vi "SubMatrixB2.vi"(0 "BCluster":T1={"Target Field, T"=1.0, "Sweep rate, T/min"=1.0, "Time btw \npoints, sec"=1.0} {"Time btw \npoints, sec" format="%.2f"; "Sweep rate, T/min" min=0.0 max=1.0 step=0.01 format="%.4f"; "Target Field, T" min=-4.0 max=4.0 step=0.1 format="%.4f"}, 1 "Instruments":T3={"Oscillator"=TRUE, "Addr 1 lock-in"=TRUE, "Addr 1 lock-in oop"=TRUE, "Addr 2 lock-in"=FALSE, "Addr 2 lock-in oop"=FALSE, "Addr 3 lock-in"=FALSE, "Addr 3 lock-in oop"=FALSE, "Voltage (Vk1)"=FALSE, "Current (Ik1)"=TRUE, "Voltage (Vk2)"=FALSE, "Current (Ik2)"=FALSE, "Voltage (Vk3)"=FALSE, "Current (Ik3)"=FALSE, "Channel 1 (Vnano1)  "=FALSE, "Channel 2 (Vnano1b)"=FALSE, "Channel 1 (Vnano2)   "=FALSE, "Channel 2 (Vnano2b)"=FALSE, "Thermometer 1 (T1)"=TRUE, "Magnetic Field (B)"=TRUE, "Capacitance (C) and Loss (L)"=FALSE}, 2 "Settings":T2={"Ring 3"=1, "Ring 2"=4, "Fixed Current mkA"=0.5, "If yes, the current is:"=enum."Radio Selection 1", "Ressitance measurements?"=TRUE, "Commute DC current?"=FALSE} {"Ring 3" items=["1 kOhm", "10 kOhm", "100 kOhm", "1 Mohm", "10 mOhm"]; "Ring 2" items=["1 kOhm", "10 kOhm", "100 kOhm", "1 Mohm", "10 MOhm"]}, 3 "Custom Folder":string, 4 "Time Stamp":timestamp) -> ()   [LabVIEW 2017]
uses:
  <vilib>/Utility/file.llb/Write To Spreadsheet File (DBL).vi
panel:
  out "Vk2ini":dbl
  out "Communication":string
  out "Current":dbl
  out "Comments":string[](array[string])
  out "ArrayBoolian":bool[][](array[boolean])
  out "Delib Time delay":i32
  out "XY Graph":cluster{dbl[], dbl[]}(graph)={[1.0, 0.8, 0.6000000000000001, 0.4000000000000001, 0.20000000000000007, 5.551115123125783e-17, -0.19999999999999996, -0.39999999999999997, -0.6, -0.8, -1.0], [0.03352775, 0.056811, 0.03911575, 0.04330675, -0.02468015, 0.011641600000000002, 0.10151450000000001, 0.12386675000000001, 0.08288825000000001, -0.00186266, -0.038650000000000004]}
  out "array for data":dbl[](array[numeric])
  in  "Ring":u16(ring) caption="Y-axis:" items=["Vg", "Vk2", "Ik2", "Vnano1", "T1", "B", "cVk2", "cIk2", "cVnano1", "cT1", "cB"]
  out "Data file:":path
  # "Lock-in Amplifiers"
  # "Temperature"
  # "SourceMeters"
  # "Nanovoltmeters"
  # "Main"
  # "(not recommended, too slow)"
  # "Magnetic Field"
  # "Capacitance & Loss"
  # "(not recommended, too slow)"
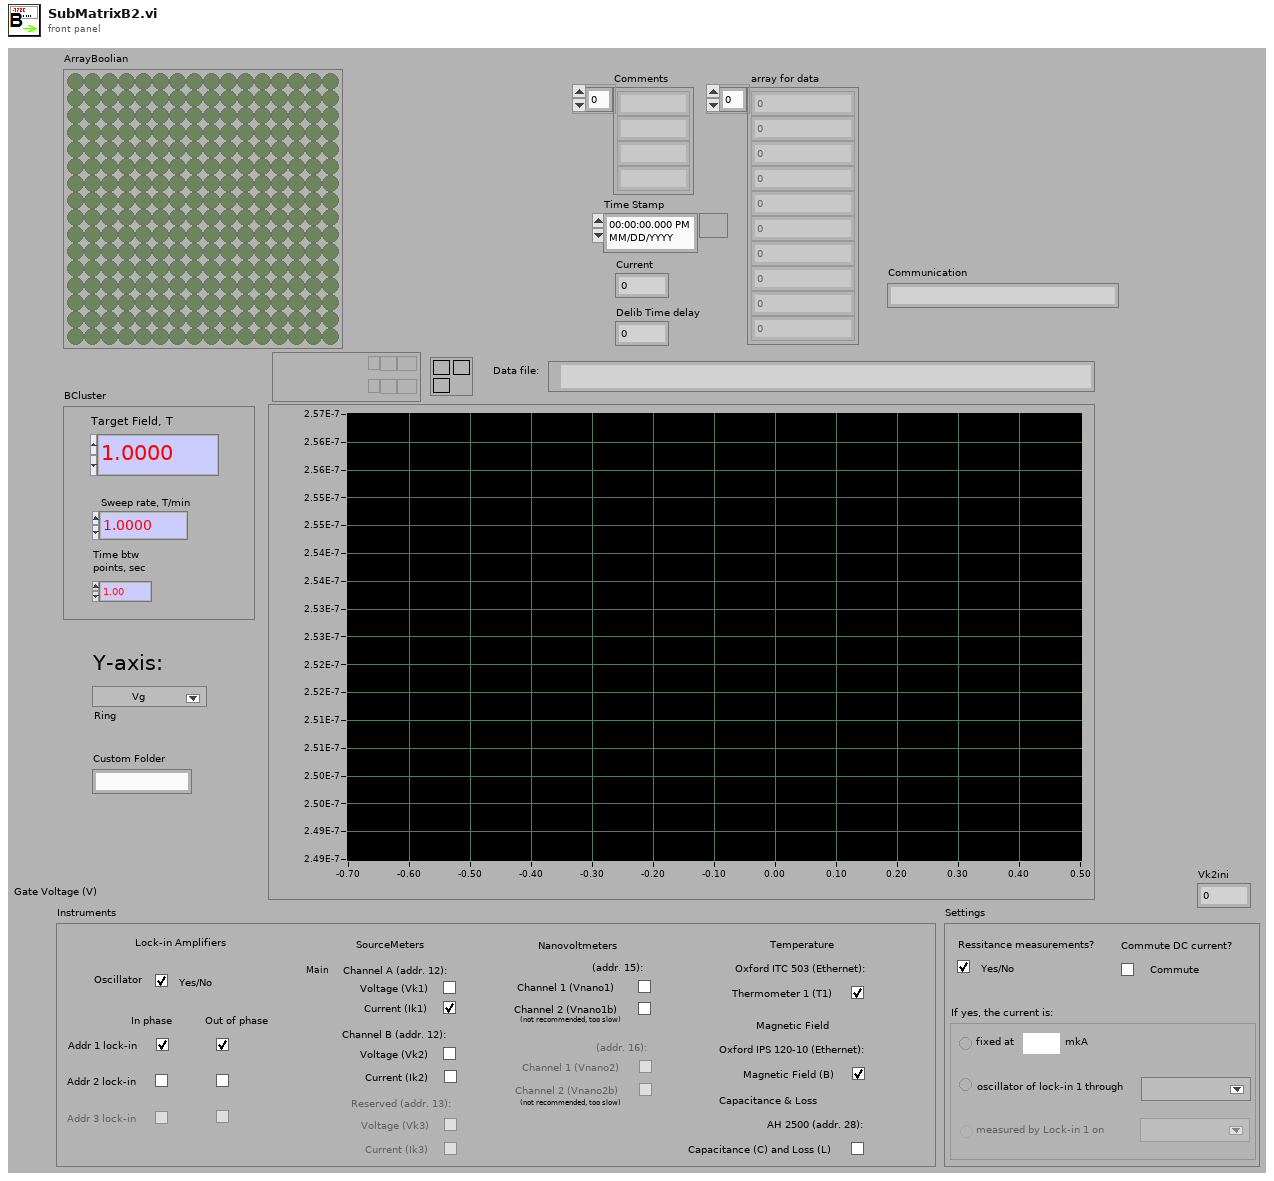
[diagram p1: front panel]
types:
  T1 = cluster{"Target Field, T":dbl, "Sweep rate, T/min":dbl, "Time btw \npoints, sec":dbl}
  T2 = cluster{"Ring 3":u16, "Ring 2":u16, "Fixed Current mkA":dbl, "If yes, the current is:":enum32{"Radio Selection 1", "Radio Selection 2", "Radio Selection 3"}, "Ressitance measurements?":bool, "Commute DC current?":bool}
  T3 = cluster{"Oscillator":bool, "Addr 1 lock-in":bool, "Addr 1 lock-in oop":bool, "Addr 2 lock-in":bool, "Addr 2 lock-in oop":bool, "Addr 3 lock-in":bool, "Addr 3 lock-in oop":bool, "Voltage (Vk1)":bool, "Current (Ik1)":bool, "Voltage (Vk2)":bool, "Current (Ik2)":bool, "Voltage (Vk3)":bool, "Current (Ik3)":bool, "Channel 1 (Vnano1)  ":bool, "Channel 2 (Vnano1b)":bool, "Channel 1 (Vnano2)   ":bool, "Channel 2 (Vnano2b)":bool, "Thermometer 1 (T1)":bool, "Magnetic Field (B)":bool, "Capacitance (C) and Loss (L)":bool}
  T4 = enum32{"Radio Selection 1", "Radio Selection 2", "Radio Selection 3"}
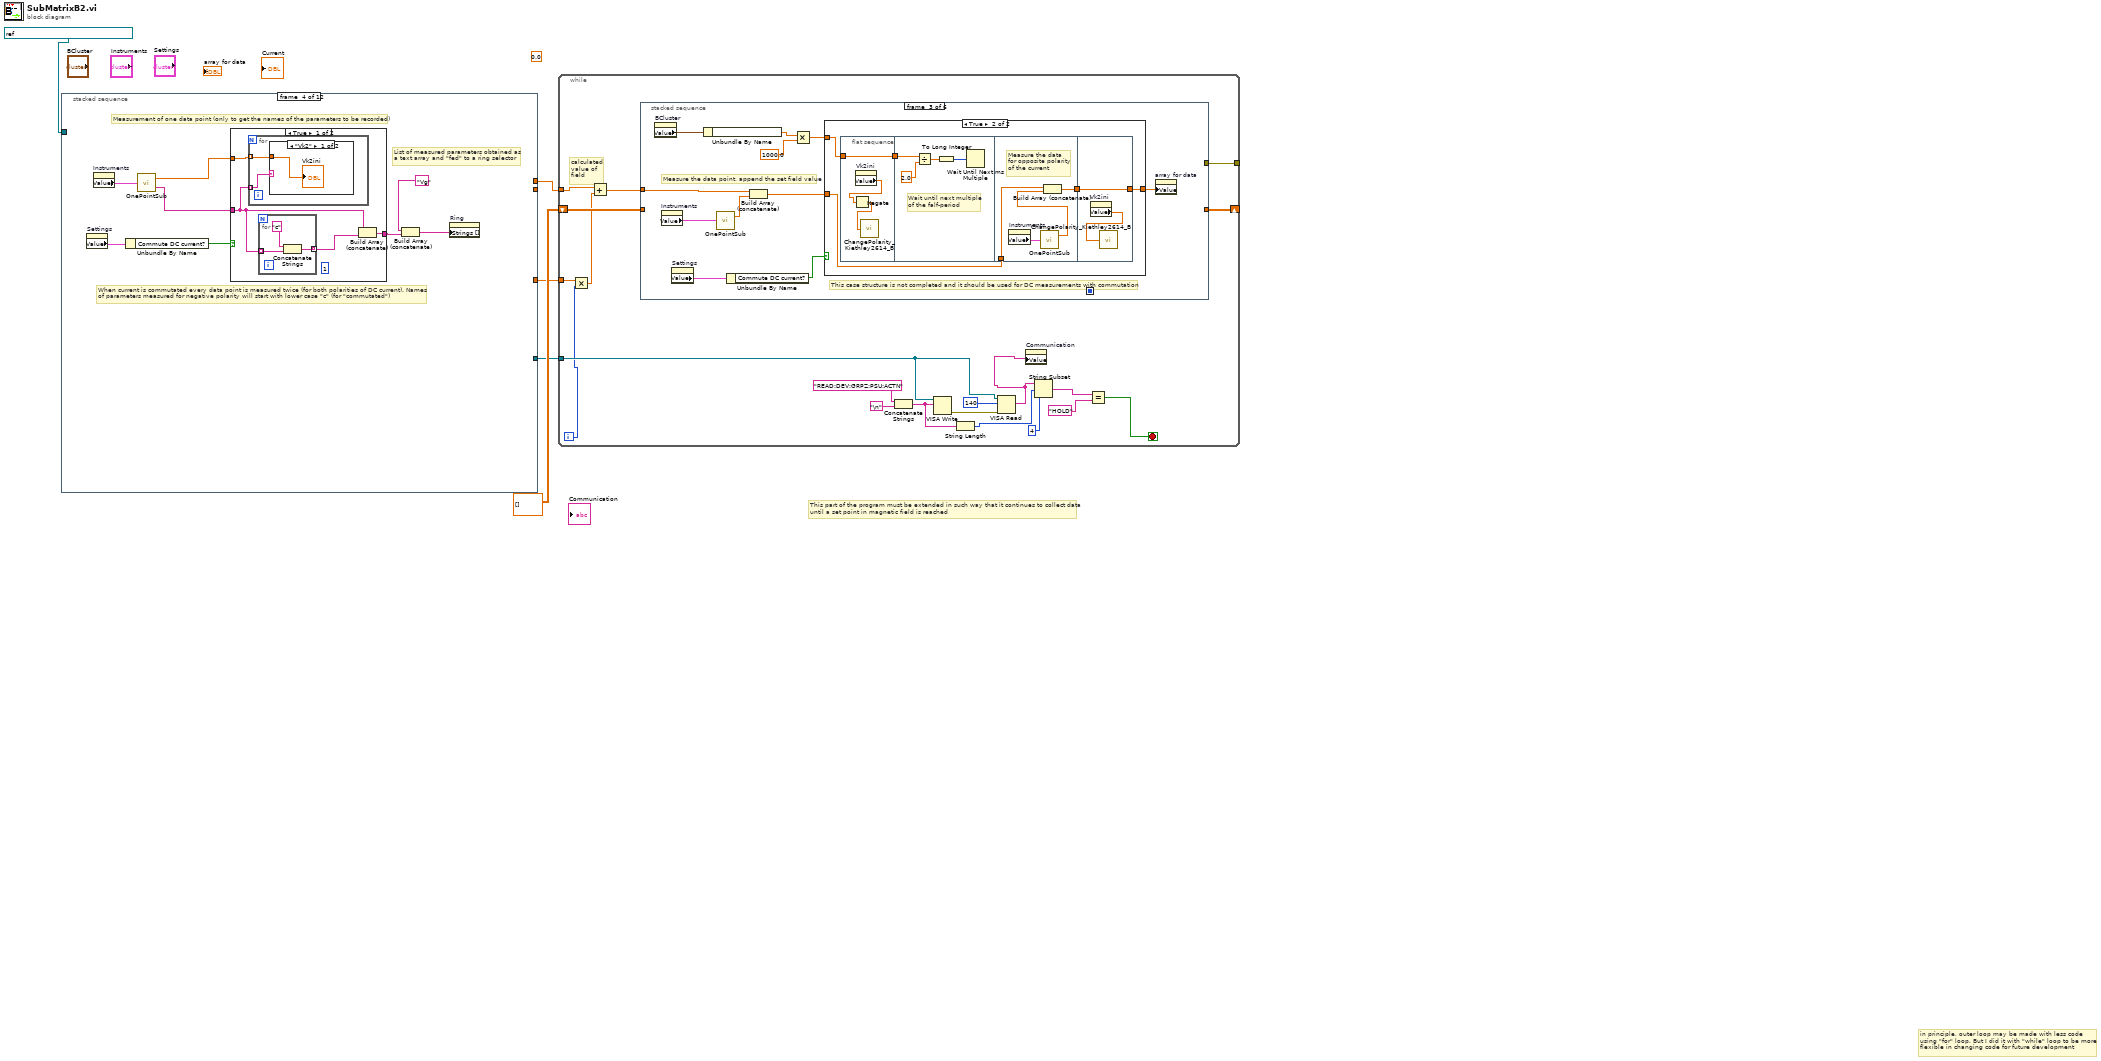
[diagram p0: block diagram]
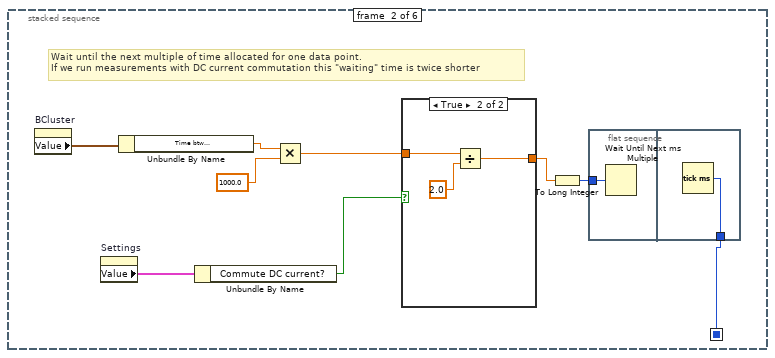
[diagram p3: hidden frame]
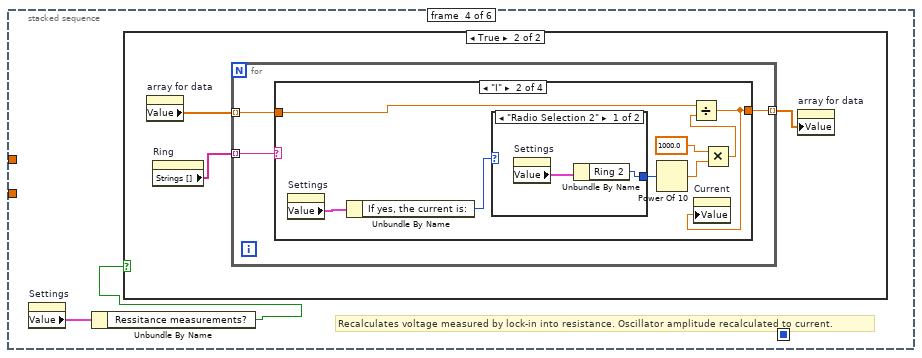
[diagram p6: hidden frame]
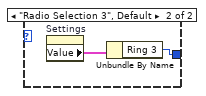
[diagram p9: hidden frame]
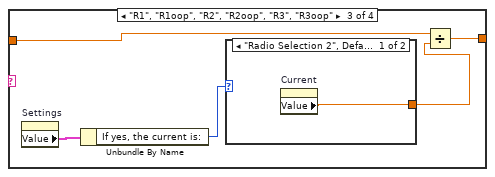
[diagram p10: hidden frame]
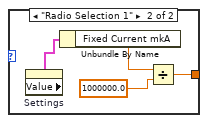
[diagram p11: hidden frame]
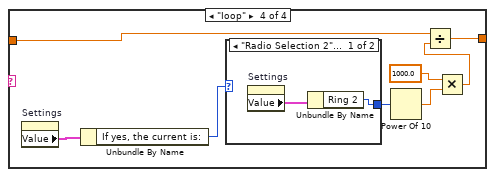
[diagram p12: hidden frame]
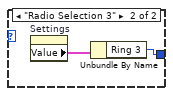
[diagram p13: hidden frame]
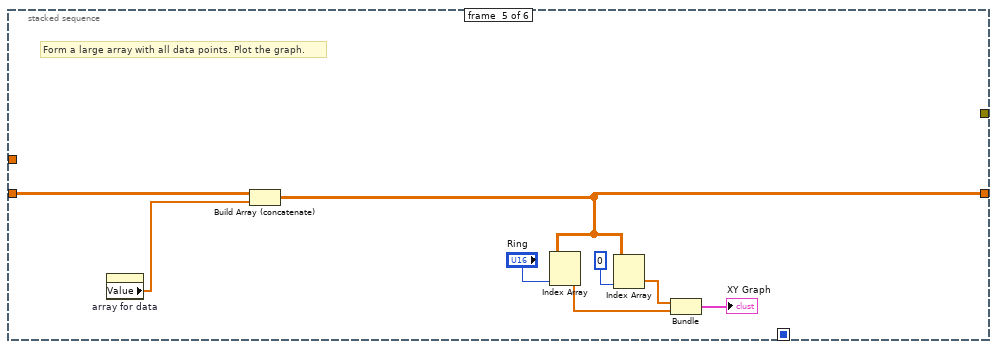
[diagram p14: hidden frame]
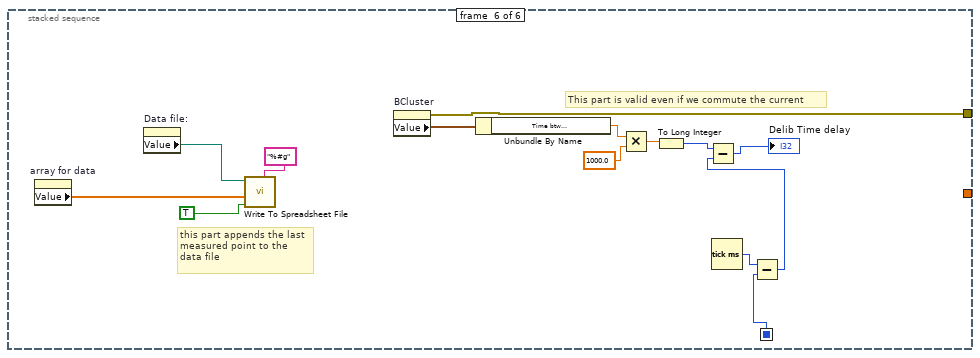
[diagram p15: hidden frame]
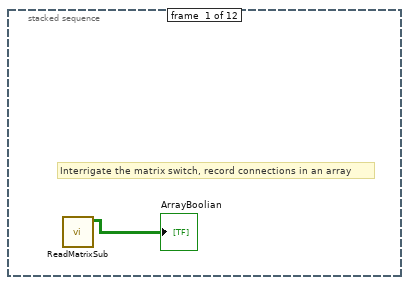
[diagram p16: hidden frame]
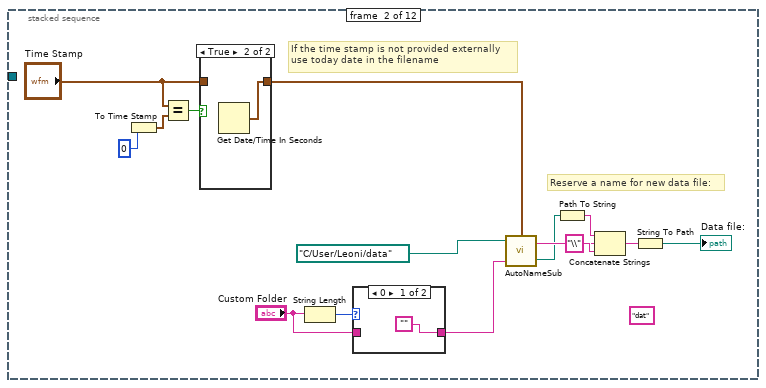
[diagram p17: hidden frame]
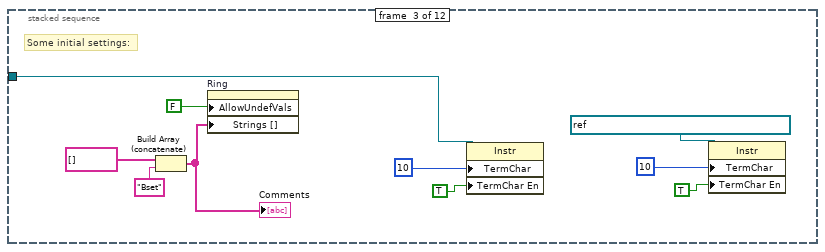
[diagram p20: hidden frame]
diagram:
  (unwired) 0.0
  # "This part of the program must be extended in such way that it continues to collect data\nuntil a set point in magnetic field is reached"
  # "in principle, outer loop may be made with less code\nusing \"for\" loop. But I did it with \"while\" loop to be more \nflexible in changing code for future development"
  n1 = stacked-sequence {
    tunnel: [_ _ _ _ _ _ _ _ _ w139 _ _] -> _
    tunnel: refnum<visa-resource-name> "TCPIP0::192.168.128.3::7020::SOCKET" ("VISA resource name") -> [_ _ w26 _ _ _ _ w100 _ w138 w174 w240]
    tunnel: [_ _ _ _ _ _ _ _ _ w138 _ _] -> w3
    tunnel: [_ _ _ _ _ _ _ _ _ w133 _ _] -> w2
    tunnel: [_ _ _ _ _ _ _ _ _ w132 _ _] -> w1
    frame #0 {
      # "Interrigate the matrix switch, record connections in an array"
      n2 = call "ReadMatrixSub.vi"() -> ("Array"=→"ArrayBoolian":bool[][])  [unwired: 9 in, 2 out]
    }
    frame #1 {
      (unwired) "dat"
      # "If the time stamp is not provided externally\nuse today date in the filename"
      # "Reserve a name for new data file:"
      n3 = To Time Stamp(1:0) -> (0:w10:timestamp)
      n4 = Equal?(x="Time Stamp", y=w10) -> (x = y?=w9:bool)
      n5 = case shown="True" w9 {
        tunnel: "Time Stamp" -> [w22 _]
        tunnel: [w22 w23] -> w7
        frame False {
        }
        frame True {
          n6 = Get Date/Time In Seconds() -> (seconds since 1Jan1904=w23:timestamp)
        }
      }
      n7 = String Length(string="Custom Folder") -> (length=w14:i32)
      n8 = case shown="0" w14 {
        tunnel: "Custom Folder" -> [_ w25]
        tunnel: ["" w25] -> w12
        frame 0 {
        }
        frame 1, Default {
        }
      }
      n9 = call "AutoNameSub.vi"("Time Stamp"=w7, "Custom Folder"=w12, "User Data Folder"=path "C:/User/Leoni/data") -> ("created path"=w20:path, "String"=w21:string)  [unwired: 1 in]
      n10 = Path To String(path=w20) -> (string=w15:string)
      n11 = Concatenate Strings(w15, "\\", w21) -> (w17:string)
      n12 = String To Path(string=w17) -> (path=→"Data file:":path)
    }
    frame #2 {
      # "Some initial settings:"
      n13 = Build Array (concatenate)(string[] [], "Bset") -> (w27:string[])
      "Comments" <- w27
      n14 = property on="Ring" class="Ring (strict)"("AllowUndefVals"=FALSE, "Strings []"=w27) -> ()  [unwired: 2 in, 2 out]
      n15 = property class="Instr"(reference=w26, "TermChar"=10, "TermChar En"=TRUE) -> ()  [unwired: 1 in, 2 out]
      n16 = property class="Instr"(reference=refnum<visa-resource-name> "TCPIP0::192.168.128.2::7020::SOCKET" ("VISA resource name"), "TermChar"=10, "TermChar En"=TRUE) -> ()  [unwired: 1 in, 2 out]
    }
    frame #3 {
      # "List of measured parameters obtained as \na text array and \"fed\" to a ring selector"
      # "When current is commutated every data point is measured twice (for both polarities of DC current). Names \nof parameters measured for negative polarity will start with lower case \"c\" (for \"commutated\")"
      # "Measurement of one data point (only to get the names of the parameters to be recorded)"
      n17 = property on="Settings" class="Clust (strict)"() -> ("Value"=w42:T2)  [unwired: 2 in, 2 out]
      n18 = property on="Instruments" class="Clust (strict)"() -> ("Value"=w40:T3)  [unwired: 2 in, 2 out]
      n19 = Unbundle By Name(w42) -> ("Commute DC current?"=w43:bool)
      n20 = call "OnePointSub.vi"("cluster"=w40) -> ("TextArray"=w41:string[], "Array"=w36:dbl[])  [unwired: 2 in]
      n21 = case shown="True" w43 {
        tunnel: w41 -> [w46 w54]
        tunnel: [w47 w54] -> w39
        tunnel: w36 -> [w45 _]
        frame True {
          (unwired) 1
          n22 = for {
            tunnel: w46 -> [w49] mode=indexing
            tunnel: w45 -> [w48] mode=indexing
            n23 = case shown="\"Vk2\"" w49 {
              tunnel: w48 -> [w50 _]
              frame "Vk2" {
                "Vk2ini" <- w50
              }
              frame Default {
              }
            }
          }
          n24 = for {
            tunnel: [w53] -> w44 mode=indexing
            tunnel: w46 -> [w51] mode=indexing
            n25 = Concatenate Strings("c", w51) -> (w53:string)
          }
          n26 = Build Array (concatenate)(w46, w44) -> (w47:string[])
        }
        frame False {
        }
      }
      n27 = Build Array (concatenate)("Vg", w39) -> (w37:string[])
      n28 = property on="Ring" class="Ring (strict)"("Strings []"=w37) -> ()  [unwired: 2 in, 2 out]
    }
    frame #4 {
      # "If resistance is not something that we are interested in, then replace \"R\" with \"V\" in all strings"
      n29 = property on="Settings" class="Clust (strict)"() -> ("Value"=w55:T2)  [unwired: 2 in, 2 out]
      n30 = Unbundle By Name(w55) -> ("Ressitance measurements?"=w56:bool)
      n31 = case shown="False" w56 {
        frame True {
        }
        frame False {
          n32 = property on="Ring" class="Ring (strict)"() -> ("Strings []"=w58:string[])  [unwired: 2 in, 2 out]
          n33 = for {
            tunnel: w58 -> [w61] mode=indexing
            tunnel: [w59] -> w57 mode=indexing
            n34 = String Subset(string=w61, length (rest)=1) -> (substring=w63:string)  [unwired: 1 in]
            n35 = Equal?(x=w63, y="R") -> (x = y?=w62:bool)
            n36 = case shown="True" w62 {
              tunnel: w61 -> [w65 w69]
              tunnel: [w65 w66] -> w59
              frame False {
              }
              frame True {
                n37 = Replace Substring(2:1, 4:"V", 5:w69) -> (1:w66:string)  [unwired: 1 in, 1 out]
              }
            }
          }
          n38 = property on="Ring" class="Ring (strict)"("Strings []"=w57) -> ()  [unwired: 2 in, 2 out]
        }
      }
    }
    frame #5 {
      # "This part makes comment line for the \ndata file. Comments are very useful for\ndouble checking that connections are \ncorrect when the data file is opened\nin Origin."
      # "Check how the oscillator is wired to the matrix switch and record connection as a comment"
      n39 = property on="Instruments" class="Clust (strict)"() -> ("Value"=w72:T3)  [unwired: 2 in, 2 out]
      n40 = property on="Comments" class="Arr (strict)"() -> ("Value"=w71:string[])  [unwired: 2 in, 2 out]
      n41 = Unbundle By Name(w72) -> ("Oscillator"=w73:bool)
      n42 = case shown="True" w73 {
        tunnel: [w74 w77] -> w70
        tunnel: w71 -> [w74 w76]
        frame False {
          # "we are not measuring oscillator from\nlock-in (address 1)"
        }
        frame True {
          (unwired) "I"
          # "This subVI takes the matrix column # (instrument\nconnection point) as an argument and finds the raw\n# (contact) to which the instrument is connected"
          # "we are  measuring oscillator"
          n43 = property on="ArrayBoolian" class="Arr (strict)"() -> ("Value"=w80:bool[][])  [unwired: 2 in, 2 out]
          n44 = GPIB Clear(3:"1") -> ()  [unwired: 1 in, 2 out]
          n45 = call "FindInstrConnect.vi"("Column #"=1, "ArrayBoolian"=w80) -> ("String"=w81:string)  [unwired: 1 in, 2 out]
          n46 = call "FindInstrConnect.vi"("Column #"=0, "ArrayBoolian"=w80) -> ("String"=w78:string)  [unwired: 1 in, 2 out]
          n47 = Concatenate Strings(w78, "-", w81) -> (w75:string)
          n48 = Build Array (concatenate)(w76, w75) -> (w77:string[])
        }
      }
      n49 = property on="Comments" class="Arr (strict)"("Value"=w70) -> ()  [unwired: 2 in, 2 out]
    }
    frame #6 {
      # "Check how the input of Lock-in 1 is wired the the matrix switch and record connection as a comment"
      n50 = property on="Instruments" class="Clust (strict)"() -> ("Value"=w87:T3)  [unwired: 2 in, 2 out]
      n51 = property on="Comments" class="Arr (strict)"() -> ("Value"=w86:string[])  [unwired: 2 in, 2 out]
      n52 = Unbundle By Name(w87) -> ("Addr 1 lock-in"=w88:bool)
      n53 = case shown="True" w88 {
        tunnel: [w89 w92] -> w85
        tunnel: w86 -> [w89 w91]
        frame False {
          # "we are not measuring oscillator from\nlock-in (address 1)"
        }
        frame True {
          (unwired) "I"
          # "This subVI takes the matrix column # (instrument\nconnection point) as an argument and finds the raw\n# (contact) to which the instrument is connected"
          # "we are  measuring Lock-In 1"
          n54 = property on="ArrayBoolian" class="Arr (strict)"() -> ("Value"=w95:bool[][])  [unwired: 2 in, 2 out]
          n55 = GPIB Clear(3:"1") -> ()  [unwired: 1 in, 2 out]
          n56 = call "FindInstrConnect.vi"("Column #"=3, "ArrayBoolian"=w95) -> ("String"=w96:string)  [unwired: 1 in, 2 out]
          n57 = call "FindInstrConnect.vi"("Column #"=2, "ArrayBoolian"=w95) -> ("String"=w93:string)  [unwired: 1 in, 2 out]
          n58 = Concatenate Strings(w93, "-", w96) -> (w90:string)
          n59 = Build Array (concatenate)(w91, w90) -> (w92:string[])
        }
      }
      n60 = property on="Comments" class="Arr (strict)"("Value"=w85) -> ()  [unwired: 2 in, 2 out]
    }
    frame #7 {
      n61 = while {
        tunnel: w100 -> [w110]
        stop <- w103 stop-if-true
        n62 = Wait (ms)(milliseconds to wait=500) -> ()  [unwired: 1 out]
        n63 = Concatenate Strings("READ:DEV:GRPZ:PSU:ACTN" ("string"), "\n") -> (w107:string)
        n64 = VISA Write(VISA resource name=w110, write buffer=w107) -> (error out=w113:errorcluster)  [unwired: 1 in, 2 out]
        n65 = String Length(string=w107) -> (length=w106:i32)
        n66 = VISA Read(VISA resource name=w110, byte count=140, error in (no error)=w113) -> (read buffer=w101:string)  [unwired: 3 out]
        n67 = property on="Communication" class="Str"("Value"=w101) -> ()  [unwired: 2 in, 2 out]
        n68 = String Subset(string=w101, offset (0)=w106, length (rest)=4) -> (substring=w105:string)
        n69 = Equal?(x=w105, y="HOLD") -> (x = y?=w103:bool)
      }
    }
    frame #8 {
      w122 = "\r"
      w121 = "\n"
      # "Both lines are recorded into\nthe data file."
      # "This part converts string array with the names of measured parameters into the line of text separated by TABs. The resulting string is\nrecorded as the first line of the data file. The second line is comments with information about conections of the instruments to particular contacts."
      n70 = property on="Ring" class="Ring (strict)"() -> ("Strings []"=w115:string[])  [unwired: 2 in, 2 out]
      n71 = property on="Comments" class="Arr (strict)"() -> ("Value"=w120:string[])  [unwired: 2 in, 2 out]
      n72 = for {
        tunnel: w115 -> [w130] mode=indexing
        shift-right: [w128] -> w118
        shift-left: "" -> [w129]
        n73 = Concatenate Strings(w129, w130, "\t") -> (w128:string)
      }
      n74 = for {
        tunnel: w120 -> [w126] mode=indexing
        shift-right: [w124] -> w123
        shift-left: "" -> [w125]
        n75 = Concatenate Strings(w125, w126, "\t") -> (w124:string)
      }
      n76 = Concatenate Strings(w118, w122, w121, w122, w121, w123, w122, w121) -> (w116:string)
      n77 = property on="Data file:" class="Path"() -> ("Value"=w114:path)  [unwired: 2 in, 2 out]
      n78 = Write to Text File(file (use dialog)=w114, text=w116) -> ()  [unwired: 2 in, 3 out]
    }
    frame #9 {
      # "Step"
      # "Read real field (persistant, if in persistance mode)"
      # "Then the table is made with all values\nof the gate voltage to be measured"
      # "rounding to 0.01 T"
      # "This part reads the status and current settings of the magnet"
      n79 = property on="BCluster" class="Clust (strict)"() -> ("Value"=w169:T1)  [unwired: 2 in, 2 out]
      n80 = Concatenate Strings("READ:DEV:GRPZ:PSU:SIG:PFLD" ("string"), "\n") -> (w159:string)
      n81 = VISA Write(VISA resource name=w138, write buffer=w159) -> (error out=w165:errorcluster)  [unwired: 1 in, 2 out]
      n82 = String Length(string=w159) -> (length=w160:i32)
      n83 = Unbundle By Name(w169) -> ("Target Field, T"=w137:dbl, "Sweep rate, T/min"=w142:dbl, "Time btw \npoints, sec"=w168:dbl)
      n84 = Number To Fractional String(number=w142) -> (F-format string=w148:string)  [unwired: 3 in]
      n85 = Concatenate Strings("SET:DEV:GRPZ:PSU:SIG:RFST:" ("string"), w148) -> (w143:string)
      n86 = VISA Read(VISA resource name=w138, byte count=140, error in (no error)=w165) -> (read buffer=w161:string)  [unwired: 3 out]
      n87 = Concatenate Strings(w143, "\n") -> (w144:string)
      n88 = Multiply(x=w142, y=w168) -> (x*y=w167:dbl)
      n89 = String Subset(string=w161, offset (0)=w160) -> (substring=w158:string)  [unwired: 1 in]
      n90 = Divide(x=w167, y=60.0) -> (x/y=w134:dbl)
      n91 = VISA Write(VISA resource name=w138, write buffer=w144) -> (error out=w147:errorcluster)  [unwired: 1 in, 2 out]
      n92 = Fract/Exp String To Number(string=w158) -> (number=w157:dbl)  [unwired: 3 in, 1 out]
      n93 = VISA Read(VISA resource name=w138, byte count=140, error in (no error)=w147) -> (read buffer=w140:string)  [unwired: 3 out]
      n94 = Number To Fractional String(number=w157, width (-)=4, precision (6)=2) -> (F-format string=w170:string)  [unwired: 1 in]
      n95 = Fract/Exp String To Number(string=w170) -> (number=w133:dbl)  [unwired: 3 in, 1 out]
      n96 = Number To Fractional String(number=w133) -> (F-format string=w155:string)  [unwired: 3 in]
      n97 = Concatenate Strings("SET:DEV:GRPZ:PSU:SIG:FSET:" ("string"), w155) -> (w150:string)
      n98 = Concatenate Strings(w150, "\n") -> (w151:string)
      n99 = VISA Write(VISA resource name=w138, write buffer=w151) -> (error out=w154:errorcluster)  [unwired: 1 in, 2 out]
      n100 = VISA Read(VISA resource name=w138, byte count=140, error in (no error)=w154) -> (read buffer=w149:string)  [unwired: 3 out]
      n101 = call "LinTableSubVI.vi"("Step"=w134, "Final"=w137, "Initial"=w133) -> ("Array"=w139:dbl[])  [unwired: 1 in]
      n102 = Subtract(x=w137, y=w133) -> (x-y=w136:dbl)
      n103 = property on="Communication" class="Str"("Value"=w140) -> ()  [unwired: 2 in, 2 out]
      n104 = property on="Communication" class="Str"("Value"=w149) -> ()  [unwired: 2 in, 2 out]
      n105 = Sign(1:w136) -> (0:w135:dbl)
      n106 = Multiply(x=w134, y=w135) -> (x*y=w132:dbl)
    }
    frame #10 {
      # "Read the status of a switch heater.\nTurn switch heater ON if needed."
      n107 = Wait (ms)(milliseconds to wait=500) -> ()  [unwired: 1 out]
      n108 = Concatenate Strings("READ:DEV:GRPZ:PSU:SIG:SWHT" ("string"), "\n") -> (w183:string)
      n109 = VISA Write(VISA resource name=w174, write buffer=w183) -> (error out=w186:errorcluster)  [unwired: 1 in, 2 out]
      n110 = String Length(string=w183) -> (length=w182:i32)
      n111 = VISA Read(VISA resource name=w174, byte count=140, error in (no error)=w186) -> (read buffer=w175:string)  [unwired: 3 out]
      n112 = String Subset(string=w175, offset (0)=w182) -> (substring=w176:string)  [unwired: 1 in]
      n113 = property on="Communication" class="Str"("Value"=w175) -> ()  [unwired: 2 in, 2 out]
      n114 = String Length(string=w176) -> (length=w179:i32)
      n115 = Decrement(x=w179) -> (x-1=w178:i32)
      n116 = String Subset(string=w176, length (rest)=w178) -> (substring=w177:string)  [unwired: 1 in]
      n117 = case shown="\"ON\"" w177 {
        tunnel: [FALSE TRUE] -> w173
        frame "OFF", Default {
        }
        frame "ON" {
        }
      }
      n118 = case shown="False" w173 {
        tunnel: w174 -> [w187 _]
        frame False {
          n119 = stacked-sequence {
            tunnel: w187 -> [w189 w195 w211 w216 _]
            frame #0 {
              # "Magnet is in a persistant mode.\nRamp the magnet to the set field."
              n120 = Concatenate Strings("SET:DEV:GRPZ:PSU:ACTN:RTOS" ("string"), "\n") -> (w191:string)
              n121 = VISA Write(VISA resource name=w189, write buffer=w191) -> (error out=w194:errorcluster)  [unwired: 1 in, 2 out]
              n122 = VISA Read(VISA resource name=w189, byte count=140, error in (no error)=w194) -> (read buffer=w188:string)  [unwired: 3 out]
              n123 = property on="Communication" class="Str"("Value"=w188) -> ()  [unwired: 2 in, 2 out]
            }
            frame #1 {
              # "Wait until the magnet reached HOLD state."
              n124 = while {
                tunnel: w195 -> [w205]
                stop <- w198 stop-if-true
                n125 = Wait (ms)(milliseconds to wait=500) -> ()  [unwired: 1 out]
                n126 = Concatenate Strings("READ:DEV:GRPZ:PSU:ACTN" ("string"), "\n") -> (w202:string)
                n127 = VISA Write(VISA resource name=w205, write buffer=w202) -> (error out=w208:errorcluster)  [unwired: 1 in, 2 out]
                n128 = String Length(string=w202) -> (length=w201:i32)
                n129 = VISA Read(VISA resource name=w205, byte count=140, error in (no error)=w208) -> (read buffer=w196:string)  [unwired: 3 out]
                n130 = property on="Communication" class="Str"("Value"=w196) -> ()  [unwired: 2 in, 2 out]
                n131 = String Subset(string=w196, offset (0)=w201, length (rest)=4) -> (substring=w200:string)
                n132 = Equal?(x=w200, y="HOLD") -> (x = y?=w198:bool)
              }
            }
            frame #2 {
              # "Turn a switch heater ON"
              n133 = Concatenate Strings("SET:DEV:GRPZ:PSU:SIG:SWHT:ON" ("string"), "\n") -> (w212:string)
              n134 = VISA Write(VISA resource name=w211, write buffer=w212) -> (error out=w215:errorcluster)  [unwired: 1 in, 2 out]
              n135 = VISA Read(VISA resource name=w211, byte count=140, error in (no error)=w215) -> (read buffer=w209:string)  [unwired: 3 out]
              n136 = property on="Communication" class="Str"("Value"=w209) -> ()  [unwired: 2 in, 2 out]
            }
            frame #3 {
              # "Wait until heater status is On"
              n137 = while {
                tunnel: w216 -> [w227]
                stop <- w219 stop-if-true
                n138 = Wait (ms)(milliseconds to wait=500) -> ()  [unwired: 1 out]
                n139 = Concatenate Strings("READ:DEV:GRPZ:PSU:SIG:SWHT" ("string"), "\n") -> (w226:string)
                n140 = VISA Write(VISA resource name=w227, write buffer=w226) -> (error out=w230:errorcluster)  [unwired: 1 in, 2 out]
                n141 = String Length(string=w226) -> (length=w225:i32)
                n142 = VISA Read(VISA resource name=w227, byte count=140, error in (no error)=w230) -> (read buffer=w217:string)  [unwired: 3 out]
                n143 = property on="Communication" class="Str"("Value"=w217) -> ()  [unwired: 2 in, 2 out]
                n144 = String Subset(string=w217, offset (0)=w225) -> (substring=w218:string)  [unwired: 1 in]
                n145 = String Length(string=w218) -> (length=w222:i32)
                n146 = Decrement(x=w222) -> (x-1=w221:i32)
                n147 = String Subset(string=w218, length (rest)=w221) -> (substring=w220:string)  [unwired: 1 in]
                n148 = case shown="\"ON\"" w220 {
                  tunnel: [FALSE TRUE] -> w219
                  frame "OFF", Default {
                  }
                  frame "ON" {
                  }
                }
              }
            }
            frame #4 {
              n149 = Wait (ms)(milliseconds to wait=10000) -> ()  [unwired: 1 out]
            }
          }
        }
        frame True {
        }
      }
    }
    frame #11 {
      n150 = property on="BCluster" class="Clust (strict)"() -> ("Value"=w257:T1)  [unwired: 2 in, 2 out]
      n151 = Unbundle By Name(w257) -> ("Target Field, T"=w238:dbl, "Sweep rate, T/min"=w241:dbl, "Time btw \npoints, sec"=w256:dbl)
      n152 = Number To Fractional String(number=w238) -> (F-format string=w252:string)  [unwired: 3 in]
      n153 = Concatenate Strings("SET:DEV:GRPZ:PSU:SIG:FSET:" ("string"), w252) -> (w247:string)
      n154 = Concatenate Strings("SET:DEV:GRPZ:PSU:ACTN:RTOS" ("string"), "\n") -> (w242:string)
      n155 = Multiply(x=w241, y=w256) -> (x*y=w255:dbl)
      n156 = Concatenate Strings(w247, "\n") -> (w248:string)
      n157 = Divide(x=w255, y=60.0) -> ()  [unwired: 1 out]
      n158 = VISA Write(VISA resource name=w240, write buffer=w248) -> (error out=w251:errorcluster)  [unwired: 1 in, 2 out]
      n159 = VISA Read(VISA resource name=w240, byte count=140, error in (no error)=w251) -> (read buffer=w246:string, error out=w237:errorcluster)  [unwired: 2 out]
      n160 = VISA Write(VISA resource name=w240, write buffer=w242, error in (no error)=w237) -> (error out=w245:errorcluster)  [unwired: 2 out]
      n161 = VISA Read(VISA resource name=w240, byte count=140, error in (no error)=w245) -> (read buffer=w239:string)  [unwired: 3 out]
      n162 = property on="Communication" class="Str"("Value"=w239) -> ()  [unwired: 2 in, 2 out]
      n163 = property on="Communication" class="Str"("Value"=w246) -> ()  [unwired: 2 in, 2 out]
    }
  }
  n164 = while {
    shift-right: [w276] -> _
    shift-left: dbl[][] [] -> [w277]
    tunnel: [w275] -> _
    tunnel: w2 -> [w262]
    tunnel: w3 -> [w265]
    tunnel: w1 -> [w260]
    i -> [w259]
    stop <- w263 stop-if-true
    # "calculated\nvalue of \nfield"
    n165 = Multiply(x=w260, y=w259) -> (x*y=w258:dbl)
    n166 = Add(x=w262, y=w258) -> (x+y=w261:dbl)
    n167 = stacked-sequence {
      seq-local: [_ w278 _ _ _ _] -> [_ _ _ _ _ w382]
      tunnel: w261 -> [_ _ w295 _ _ _]
      tunnel: w277 -> [_ _ _ _ w368 _]
      tunnel: [_ _ _ _ w366 _] -> w276
      tunnel: [_ _ _ _ _ w374] -> w275
      frame #0 {
        # "send new Vg value to main Keithley 2400"
      }
      frame #1 {
        # "Wait until the next multiple of time allocated for one data point.\nIf we run measurements with DC current commutation this \"waiting\" time is twice shorter"
        n168 = property on="BCluster" class="Clust (strict)"() -> ("Value"=w286:T1)  [unwired: 2 in, 2 out]
        n169 = property on="Settings" class="Clust (strict)"() -> ("Value"=w283:T2)  [unwired: 2 in, 2 out]
        n170 = Unbundle By Name(w286) -> ("Time btw \npoints, sec"=w285:dbl)
        n171 = Unbundle By Name(w283) -> ("Commute DC current?"=w282:bool)
        n172 = Multiply(x=w285, y=1000.0) -> (x*y=w281:dbl)
        n173 = case shown="True" w282 {
          tunnel: w281 -> [w289 w291]
          tunnel: [w289 w290] -> w280
          frame False {
          }
          frame True {
            n174 = Divide(x=w291, y=2.0) -> (x/y=w290:dbl)
          }
        }
        n175 = To Long Integer(number=w280) -> (32bit integer=w279:i32)
        n176 = flat-sequence {
          tunnel: w279 -> [w287]
          tunnel: [w288] -> w278
          frame #0 {
            n177 = Wait Until Next ms Multiple(millisecond multiple=w287) -> ()  [unwired: 1 out]
          }
          frame #1 {
            n178 = Tick Count (ms)() -> (millisecond timer value=w288:u32)
          }
        }
      }
      frame #2 {
        # "This case structure is not completed and it should be used for DC measurements with commutation"
        # "Measure the data point, append the set field value"
        n179 = property on="BCluster" class="Clust (strict)"() -> ("Value"=w303:T1)  [unwired: 2 in, 2 out]
        n180 = property on="Instruments" class="Clust (strict)"() -> ("Value"=w297:T3)  [unwired: 2 in, 2 out]
        n181 = property on="Settings" class="Clust (strict)"() -> ("Value"=w300:T2)  [unwired: 2 in, 2 out]
        n182 = Unbundle By Name(w303) -> ("Time btw \npoints, sec"=w302:dbl)
        n183 = call "OnePointSub.vi"("cluster"=w297) -> ("Array"=w296:dbl[])  [unwired: 2 in, 1 out]
        n184 = Unbundle By Name(w300) -> ("Commute DC current?"=w299:bool)
        n185 = Build Array (concatenate)(w295, w296) -> (w294:dbl[])
        n186 = Multiply(x=w302, y=1000.0) -> (x*y=w298:dbl)
        n187 = case shown="True" w299 {
          tunnel: w298 -> [_ w309]
          tunnel: [w304 w306] -> w293
          tunnel: w294 -> [w304 w307]
          frame False {
          }
          frame True {
            n188 = flat-sequence {
              tunnel: w309 -> [w312]
              tunnel: [w312] -> w308
              tunnel: w308 -> [w315]
              tunnel: w307 -> [w318]
              tunnel: [w317] -> w305
              tunnel: [w322] -> w306
              tunnel: w305 -> [w322]
              frame #0 {
                n189 = property on="Vk2ini" class="DigNum (strict)"() -> ("Value"=w310:dbl)  [unwired: 2 in, 2 out]
                n190 = Negate(x=w310) -> (-x=w311:dbl)
                n191 = call "ChangePolarity_Kiethley2614_B.vi"("Voltage (sourse)"=w311) -> ()  [unwired: 1 in]
              }
              frame #1 {
                # "Wait until next multiple\nof the falf-period"
                n192 = Divide(x=w315, y=2.0) -> (x/y=w313:dbl)
                n193 = To Long Integer(number=w313) -> (32bit integer=w314:i32)
                n194 = Wait Until Next ms Multiple(millisecond multiple=w314) -> ()  [unwired: 1 out]
              }
              frame #2 {
                # "Measure the data\nfor opposite polarity\nof the current"
                n195 = property on="Instruments" class="Clust (strict)"() -> ("Value"=w320:T3)  [unwired: 2 in, 2 out]
                n196 = call "OnePointSub.vi"("cluster"=w320) -> ("Array"=w319:dbl[])  [unwired: 2 in, 1 out]
                n197 = Build Array (concatenate)(w318, w319) -> (w317:dbl[])
              }
              frame #3 {
                n198 = property on="Vk2ini" class="DigNum (strict)"() -> ("Value"=w321:dbl)  [unwired: 2 in, 2 out]
                n199 = call "ChangePolarity_Kiethley2614_B.vi"("Voltage (sourse)"=w321) -> ()  [unwired: 1 in]
              }
            }
          }
        }
        n200 = property on="array for data" class="Arr (strict)"("Value"=w293) -> ()  [unwired: 2 in, 2 out]
      }
      frame #3 {
        # "Recalculates voltage measured by lock-in into resistance. Oscillator amplitude recalculated to current."
        n201 = property on="Settings" class="Clust (strict)"() -> ("Value"=w324:T2)  [unwired: 2 in, 2 out]
        n202 = Unbundle By Name(w324) -> ("Ressitance measurements?"=w323:bool)
        n203 = case shown="True" w323 {
          frame False {
          }
          frame True {
            n204 = property on="array for data" class="Arr (strict)"() -> ("Value"=w326:dbl[])  [unwired: 2 in, 2 out]
            n205 = property on="Ring" class="Ring (strict)"() -> ("Strings []"=w327:string[])  [unwired: 2 in, 2 out]
            n206 = for {
              tunnel: w327 -> [w330] mode=indexing
              tunnel: w326 -> [w329] mode=indexing
              tunnel: [w328] -> w325 mode=indexing
              n207 = case shown="\"I\"" w330 {
                tunnel: w329 -> [w331 w334 w346 w356]
                tunnel: [w331 w332 w345 w355] -> w328
                frame "False", Default {
                }
                frame "I" {
                  n208 = property on="Settings" class="Clust (strict)"() -> ("Value"=w339:T2)  [unwired: 2 in, 2 out]
                  n209 = Unbundle By Name(w339) -> ("If yes, the current is:"=w338:T4)
                  n210 = case shown="\"Radio Selection 2\"" w338 {
                    tunnel: [w340 w342] -> w333
                    frame "Radio Selection 2" {
                      n211 = property on="Settings" class="Clust (strict)"() -> ("Value"=w341:T2)  [unwired: 2 in, 2 out]
                      n212 = Unbundle By Name(w341) -> ("Ring 2"=w340:u16)
                    }
                    frame "Radio Selection 3", Default {
                      n213 = property on="Settings" class="Clust (strict)"() -> ("Value"=w343:T2)  [unwired: 2 in, 2 out]
                      n214 = Unbundle By Name(w343) -> ("Ring 3"=w342:u16)
                    }
                  }
                  n215 = Power Of 10(x=w333) -> (10^x=w337:dbl)
                  n216 = Multiply(x=1000.0, y=w337) -> (x*y=w335:dbl)
                  n217 = Divide(x=w334, y=w335) -> (x/y=w332:dbl)
                  n218 = property on="Current" class="DigNum (strict)"("Value"=w332) -> ()  [unwired: 2 in, 2 out]
                }
                frame "R1", "R1oop", "R2", "R2oop", "R3", "R3oop" {
                  n219 = property on="Settings" class="Clust (strict)"() -> ("Value"=w348:T2)  [unwired: 2 in, 2 out]
                  n220 = Unbundle By Name(w348) -> ("If yes, the current is:"=w347:T4)
                  n221 = case shown="\"Radio Selection 2\", Default" w347 {
                    tunnel: [w349 w352] -> w344
                    frame "Radio Selection 2", Default {
                      n222 = property on="Current" class="DigNum (strict)"() -> ("Value"=w349:dbl)  [unwired: 2 in, 2 out]
                    }
                    frame "Radio Selection 1" {
                      n223 = property on="Settings" class="Clust (strict)"() -> ("Value"=w353:T2)  [unwired: 2 in, 2 out]
                      n224 = Unbundle By Name(w353) -> ("Fixed Current mkA"=w351:dbl)
                      n225 = Divide(x=w351, y=1000000.0) -> (x/y=w352:dbl)
                    }
                  }
                  n226 = Divide(x=w346, y=w344) -> (x/y=w345:dbl)
                }
                frame "Ioop" {
                  n227 = property on="Settings" class="Clust (strict)"() -> ("Value"=w361:T2)  [unwired: 2 in, 2 out]
                  n228 = Unbundle By Name(w361) -> ("If yes, the current is:"=w360:T4)
                  n229 = case shown="\"Radio Selection 2\", Default" w360 {
                    tunnel: [w362 w364] -> w354
                    frame "Radio Selection 2", Default {
                      n230 = property on="Settings" class="Clust (strict)"() -> ("Value"=w363:T2)  [unwired: 2 in, 2 out]
                      n231 = Unbundle By Name(w363) -> ("Ring 2"=w362:u16)
                    }
                    frame "Radio Selection 3" {
                      n232 = property on="Settings" class="Clust (strict)"() -> ("Value"=w365:T2)  [unwired: 2 in, 2 out]
                      n233 = Unbundle By Name(w365) -> ("Ring 3"=w364:u16)
                    }
                  }
                  n234 = Power Of 10(x=w354) -> (10^x=w359:dbl)
                  n235 = Multiply(x=1000.0, y=w359) -> (x*y=w357:dbl)
                  n236 = Divide(x=w356, y=w357) -> (x/y=w355:dbl)
                }
              }
            }
            n237 = property on="array for data" class="Arr (strict)"("Value"=w325) -> ()  [unwired: 2 in, 2 out]
          }
        }
      }
      frame #4 {
        # "Form a large array with all data points. Plot the graph."
        n238 = property on="array for data" class="Arr (strict)"() -> ("Value"=w367:dbl[])  [unwired: 2 in, 2 out]
        n239 = Build Array (concatenate)(w368, w367) -> (w366:dbl[][])
        n240 = Index Array(array=w366, index (col)="Ring") -> (element=w373:dbl[])  [unwired: 1 in]
        n241 = Index Array(array=w366, index (col)=0) -> (element=w371:dbl[])  [unwired: 1 in]
        n242 = Bundle(w371, w373) -> (→"XY Graph":cluster{dbl[], dbl[]})  [unwired: 1 in]
      }
      frame #5 {
        # "This part is valid even if we commute the current"
        # "this part appends the last\nmeasured point to the \ndata file"
        n243 = property on="array for data" class="Arr (strict)"() -> ("Value"=w387:dbl[])  [unwired: 2 in, 2 out]
        n244 = property on="Data file:" class="Path"() -> ("Value"=w385:path)  [unwired: 2 in, 2 out]
        n245 = call-poly <vilib>:"Write To Spreadsheet File.vi"("format (%.3f)"="%#g", "append to file? (new file:F)"=TRUE, "1D data"=w387, "file path (dialog if empty)"=w385) -> ()  [unwired: 4 in, 1 out]
        n246 = property on="BCluster" class="Clust (strict)"() -> (error out=w374:errorcluster, "Value"=w381:T1)  [unwired: 2 in, 1 out]
        n247 = Unbundle By Name(w381) -> ("Time btw \npoints, sec"=w380:dbl)
        n248 = Multiply(x=w380, y=1000.0) -> (x*y=w378:dbl)
        n249 = To Long Integer(number=w378) -> (32bit integer=w377:i32)
        n250 = Tick Count (ms)() -> (millisecond timer value=w383:u32)
        n251 = Subtract(x=w383, y=w382) -> (x-y=w375:u32)
        n252 = Subtract(x=w377, y=w375) -> (x-y=→"Delib Time delay":u32)
      }
    }
    n253 = Concatenate Strings("READ:DEV:GRPZ:PSU:ACTN" ("string"), "\n") -> (w271:string)
    n254 = VISA Write(VISA resource name=w265, write buffer=w271) -> (error out=w266:errorcluster)  [unwired: 1 in, 2 out]
    n255 = String Length(string=w271) -> (length=w272:i32)
    n256 = VISA Read(VISA resource name=w265, byte count=140, error in (no error)=w266) -> (read buffer=w274:string)  [unwired: 3 out]
    n257 = property on="Communication" class="Str"("Value"=w274) -> ()  [unwired: 2 in, 2 out]
    n258 = String Subset(string=w274, offset (0)=w272, length (rest)=4) -> (substring=w273:string)
    n259 = Equal?(x=w273, y="HOLD") -> (x = y?=w263:bool)
  }
